vi "Read Numeric Normal.vi"(0 "VISA resource name":refnum<visa-resource-name>, 9 "Mode (0: Normal)":u16(ring) items=["Normal", "Harmonics"], 11 "error in (no error)":errorcluster) -> (4 "VISA resource name out":refnum<visa-resource-name>, 6 "Read Strings":string, 8 "Measure":dbl[](array[numeric]) format="%^.3e", 15 "error out":errorcluster)   [LabVIEW 2014, in "Yokogawa.lvlib" / "Yokogawa PZ4000.lvlib"]
doc: "This VI reads the Measure Value from the PZ4000 series."
uses:
  Yokogawa PZ4000.lvlib
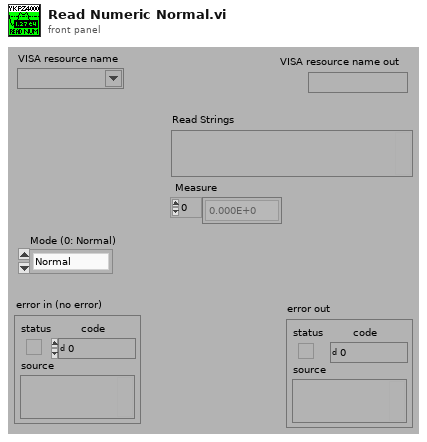
[diagram p1: front panel]
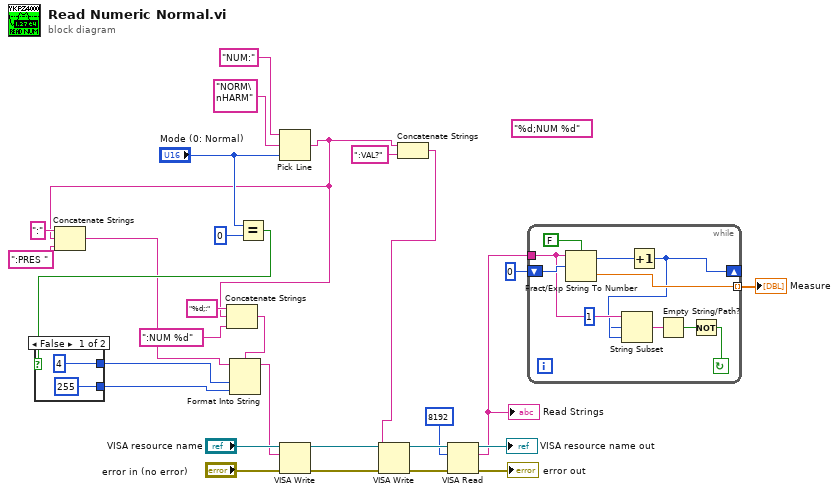
[diagram p0: block diagram]
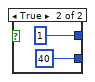
[diagram p2: hidden frame]
diagram:
  (unwired) "%d;NUM %d"
  n1 = Equal?(x="Mode (0: Normal)", y=u16 0) -> (x = y?=w10:bool)
  n2 = case shown="False" w10 {
    tunnel: [4 1] -> w12
    tunnel: [255 40] -> w11
    frame False {
    }
    frame True {
    }
  }
  n3 = Pick Line(string ("")="NUM:", multi-line string="NORM\nHARM", line index="Mode (0: Normal)") -> (output string=w3:string)
  n4 = Concatenate Strings(":" ("string"), w3, ":PRES ") -> (w5:string)
  n5 = Concatenate Strings("%d;:" ("string"), w3, ":NUM %d") -> (w1:string)
  n6 = Format Into String(format string=w1, initial string=w5, w12, w11) -> (resulting string=w17:string)  [unwired: 1 in, 1 out]
  n7 = VISA Write(VISA resource name="VISA resource name", write buffer=w17, error in (no error)="error in (no error)") -> (VISA resource name out=w20:refnum<visa-resource-name>, error out=w18:errorcluster)  [unwired: 1 out]
  n8 = Concatenate Strings(w3, ":VAL?" ("string")) -> (w8:string)
  n9 = VISA Write(VISA resource name=w20, write buffer=w8, error in (no error)=w18) -> (VISA resource name out=w28:refnum<visa-resource-name>, error out=w29:errorcluster)  [unwired: 1 out]
  n10 = VISA Read(VISA resource name=w28, byte count=u32 8192 ("ÊÞ²Ä¶³ÝÄi0j"), error in (no error)=w29) -> (VISA resource name out=→"VISA resource name out":refnum<visa-resource-name>, read buffer=w24:string, error out=→"error out":errorcluster)  [unwired: 1 out]
  "Read Strings" <- w24
  n11 = while {
    tunnel: [w42] -> w23 mode=indexing
    shift-left: 0 -> [w43]
    shift-right: [w36] -> _
    tunnel: w24 -> [w41]
    stop <- w37 continue-if-true
    n12 = Fract/Exp String To Number(use system decimal point (T)=FALSE ("¼½ÃÑ10i¬_ðgp(T)"), string=w41, offset=w43) -> (offset past number=w35:i32, number=w42:dbl)  [unwired: 1 in]
    n13 = Increment(x=w35) -> (x+1=w36:i32)
    n14 = String Subset(string=w41, offset (0)=w36, length (rest)=1) -> (substring=w39:string)
    n15 = Empty String/Path?(string/path=w39) -> (empty?=w38:bool)
    n16 = Not(x=w38) -> (.not. x?=w37:bool)
  }
  "Measure" <- w23
